vi "padString.vi"(9 "pad":string="-", 10 "String":string="---", 11 "length":i32=3) -> (2 "resultString":string="-----------------------------------------------")   [LabVIEW 2015]
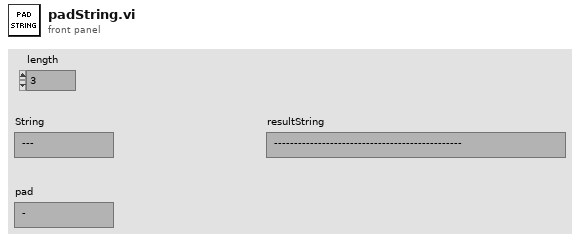
[diagram p1: front panel]
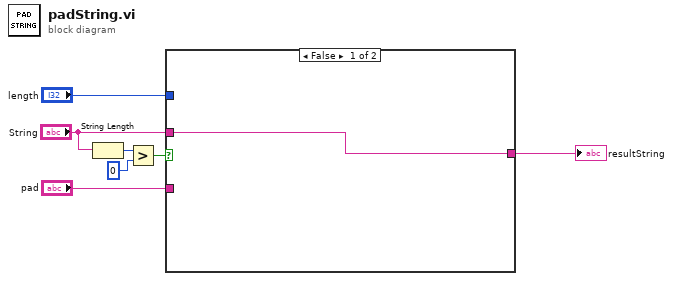
[diagram p0: block diagram]
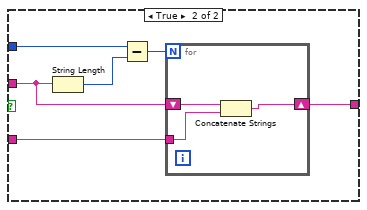
[diagram p2: hidden frame]
diagram:
  n1 = String Length(string="String") -> (length=w2:i32)
  n2 = Greater?(x=w2, y=0) -> (0:w3:bool)
  n3 = case shown="False" w3 {
    tunnel: "length" -> [_ w13]
    tunnel: "pad" -> [_ w11]
    tunnel: "String" -> [w8 w10]
    tunnel: [w8 w9] -> w5
    frame False {
    }
    frame True {
      n4 = String Length(string=w10) -> (length=w12:i32)
      n5 = Subtract(x=w13, y=w12) -> (x-y=w14:i32)
      n6 = for {
        N: w14 -> [_]
        tunnel: w11 -> [w17]
        shift-right: [w16] -> w9
        shift-left: w10 -> [w15]
        n7 = Concatenate Strings(w15, w17) -> (w16:string)
      }
    }
  }
  "resultString" <- w5
